vi "Read I32.vi"(8 "error in (no error)":errorcluster, 9 "element data type":i32, 10 "Tag Name":string, 11 "Current Value Table in":refnum<class "Current Value Table.lvclass">) -> (0 "error out":errorcluster, 2 "value":i32, 3 "Current Value Table out":refnum<class "Current Value Table.lvclass">)   [LabVIEW 2024, in "Current Value Table.lvlib" / "Current Value Table.lvclass"]
uses:
  Current Value Table.lvclass
  CVT_I32/CVT_I32.lvclass
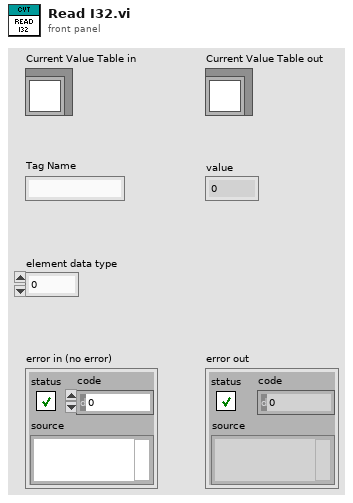
[diagram p1: front panel]
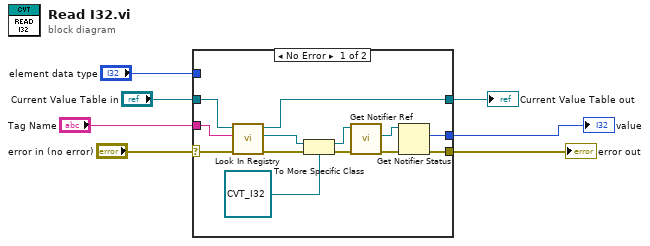
[diagram p0: block diagram]
diagram:
  n1 = case shown="No Error" "error in (no error)" {
    selector: "error in (no error)" -> [w17 w22]
    tunnel: [w9 w22] -> w6
    tunnel: [w18 w21] -> w4
    tunnel: "Current Value Table in" -> [w19 w21]
    tunnel: "element data type" -> [_ _]
    tunnel: "Tag Name" -> [w20 _]
    tunnel: [w10 _] -> w1
    frame No Error {
      n2 = call-dynamic "Look In Registry.vi"("error in (no error)"=w17, "Tag Name"=w20, "Current Value Table in"=w19) -> ("error out"=w14:errorcluster, "CVT_Item out"=w16:refnum<class "iCVT_Item.lvclass">, "Current Value Table out"=w18:refnum<class "Current Value Table.lvclass">)  [unwired: 5 in, 1 out]
      n3 = To More Specific Class(target class=refnum<class "CVT_I32.lvclass"> refnum ("Current Value Table.lvlib:CVT_I32.lvclass"), reference=w16, error in=w14) -> (specific class reference=w13:refnum<class "CVT_I32.lvclass">, error out=w12:errorcluster)
      n4 = call-dynamic "Get Notifier Ref.vi"("error in (no error)"=w12, "CVT_I32 in"=w13) -> ("error out"=w8:errorcluster, "notifier out"=w11:refnum<notifier>)  [unwired: 7 in, 1 out]
      n5 = Get Notifier Status(notifier=w11, error in (no error)=w8) -> (current notification=w10:i32, error out=w9:errorcluster)  [unwired: 3 out]
    }
    frame Error {
    }
  }
  "error out" <- w6
  "Current Value Table out" <- w4
  "value" <- w1
